vi "Eagle Command Stream Server.vi"(9 "RT Status":refnum<vi>, 10 "StatusRefs":T1, 11 "Controller IP":string="192.168.1.199") -> ()   [LabVIEW 2015]
uses:
  Controls/RT Status Refs.ctl
  Controls/LP Status typedef.ctl
  Controls/BELKIN RT State.ctl
  IP Dev Area/IP results.ctl
  Robo Team Engine Command.ctl
  RT Controls/Generic instruction typedef.ctl
  RT Controls/RT Streamer Ack element.ctl
  Controls/Eagle Green Cordinates.ctl
  <vilib>/vision/Image Controls.llb/IMAQ Image.ctl
  <vilib>/dex/Flush And Wait Empty Condition.ctl
  Controls/Command Typedef.ctl
  Robo Team Globals.vi
  GUI/Host Globals.vi
  <resource>/objmgr/ni.dex.rc
panel:
  out "XY Graph":cluster{"X Cord":u16[], "Y Cord":u16[]}(graph)
  out "Close":bool
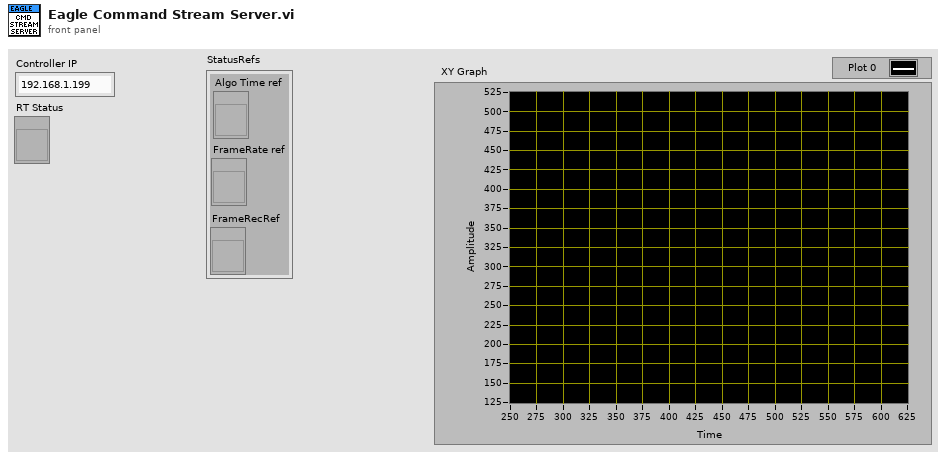
[diagram p1: front panel]
types:
  T1 = typedef "RT Status Refs.ctl" = cluster{"Algo Time ref":refnum<vi>, "FrameRate ref":refnum<vi>, "FrameRecRef":refnum<vi>}
  T2 = typedef "Generic instruction typedef.ctl" = cluster{"CMD":string, "Data":variant}
  T3 = typedef "Robo Team Engine Command.ctl" = cluster{"Command":string, "Data":variant, "Error":errorcluster, "Timeout":i32}
  T4 = typedef "Eagle Green Cordinates.ctl" = cluster{"X Cord":u16[], "Y Cord":u16[]}
  T5 = typedef "LP Status typedef.ctl" = cluster{"FrameRate":dbl, "AlgoTime":dbl, "FrameRec":u16, "System State":T6, "IP Results":T7, "SimulationMode":bool, "RotateImage":bool}
  T6 = typedef "BELKIN RT State.ctl" = enum16{"Initialize", "BIT", "Warm Up", "Eye Location", "Find Limbus", "Eye Track", "Fire", "Treatment Complete", "Shut Down", "Error"}
  T7 = typedef "IP results.ctl" = cluster{"X":u16, "Y":u16, "A":dbl, "B":dbl, "Grade":u16, "Frame#":u16}
  T8 = typedef "RT Streamer Ack element.ctl" = cluster{"Data":variant, "CMD":string, "error":errorcluster}
  T9 = typedef "IMAQ Image.ctl" = refnum<image>
  T10 = typedef "Command Typedef.ctl" = cluster{"CMD":T6, "Data":variant}
  T11 = typedef "Robo System State Refs.ctl" = cluster{"Engage Motor":refnum<vi>, "Auto Level":refnum<vi>, "IMU led":refnum<vi>, "Evaluate Enable":refnum<vi>, "Motor Led":refnum<vi>, "Error Descript":refnum<vi>, "Error Led":refnum<vi>, "Error":refnum<vi>}
  T12 = typedef "Flush And Wait Empty Condition.ctl" = u8
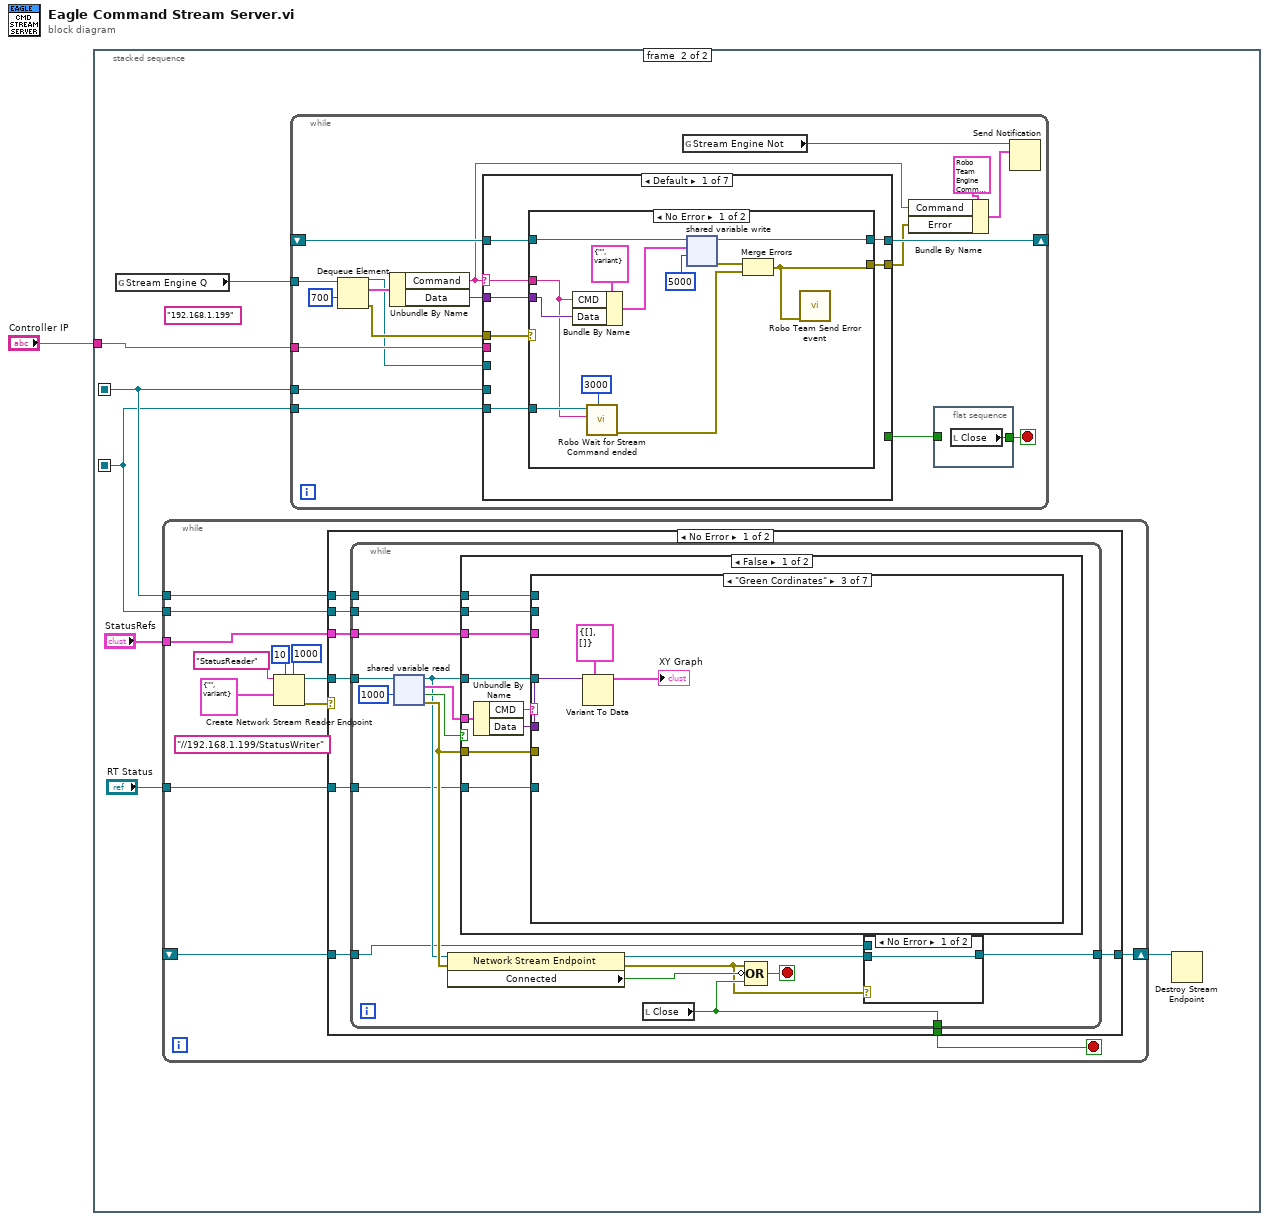
[diagram p0: block diagram]
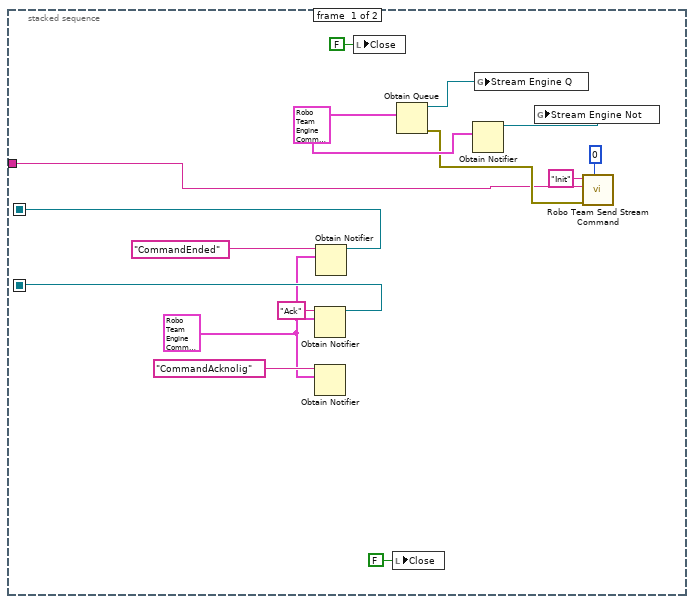
[diagram p2: hidden frame]
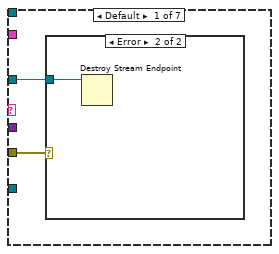
[diagram p4: hidden frame]
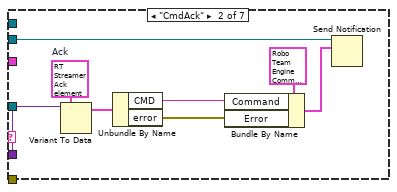
[diagram p6: hidden frame]
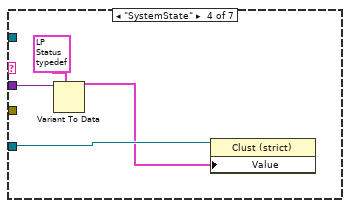
[diagram p7: hidden frame]
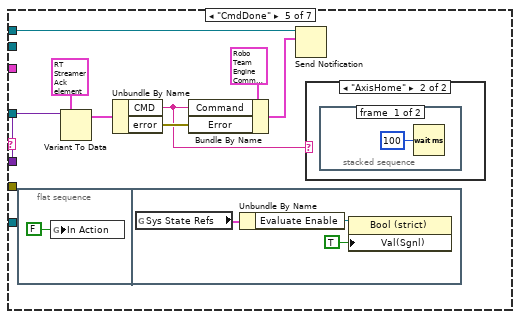
[diagram p8: hidden frame]
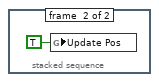
[diagram p10: hidden frame]
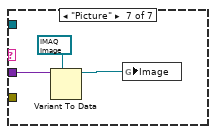
[diagram p12: hidden frame]
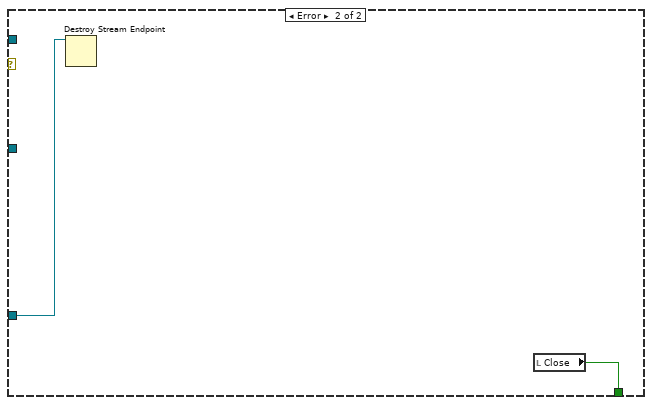
[diagram p14: hidden frame]
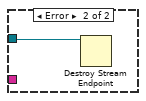
[diagram p15: hidden frame]
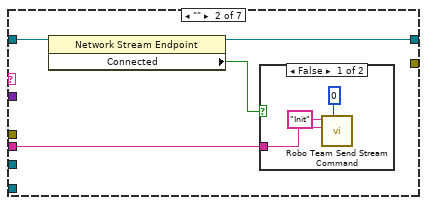
[diagram p16: hidden frame]
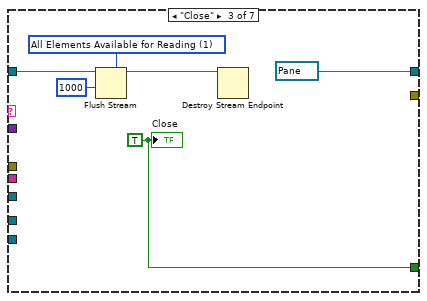
[diagram p18: hidden frame]
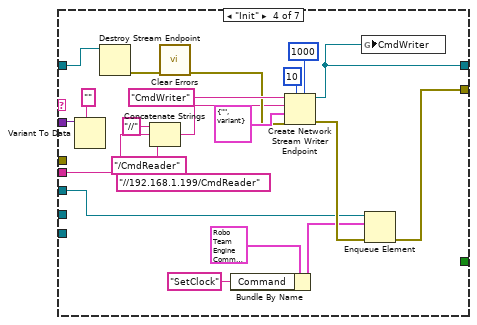
[diagram p19: hidden frame]
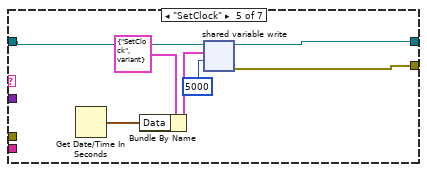
[diagram p20: hidden frame]
diagram:
  n1 = stacked-sequence {
    seq-local: [w14 _] -> [_ w22]
    seq-local: [w12 _] -> [_ w21]
    tunnel: "Controller IP" -> [w2 w18]
    frame #0 {
      w8 = T3 {"Command"="", "Data"=variant, "Error"={"status"=FALSE, "code"=0, "source"=""}, "Timeout"=0} ("notification")
      w11 = T3 {"Command"="", "Data"=variant, "Error"={"status"=FALSE, "code"=0, "source"=""}, "Timeout"=0}
      n2 = Obtain Notifier(name (unnamed)="Ack", notification data type=w11) -> (notifier out=w12:refnum<notifier>)  [unwired: 2 in, 2 out]
      n3 = Obtain Notifier(name (unnamed)="CommandAcknolig", notification data type=w11) -> ()  [unwired: 2 in, 3 out]
      n4 = Obtain Notifier(name (unnamed)="CommandEnded", notification data type=w11) -> (notifier out=w14:refnum<notifier>)  [unwired: 2 in, 2 out]
      n5 = local write "Close"(FALSE ("Close")) -> ()
      n6 = local write "Close"(FALSE ("Close")) -> ()
      n7 = Obtain Queue(element data type=w8) -> (queue out=w7:refnum<queue>, error out=w3:errorcluster)  [unwired: 4 in, 1 out]
      n8 = Obtain Notifier(notification data type=w8) -> (notifier out=w6:refnum<notifier>)  [unwired: 3 in, 2 out]
      n9 = global write "Robo Team Globals.vi" "Stream Engine Q"(w7) -> ()
      n10 = global write "Robo Team Globals.vi" "Stream Engine Not"(w6) -> ()
      n11 = call "Robo Team Send Stream Command.vi"("timeout in ms (0)"=0 ("timeout in ms (5000)"), "error in (no error)"=w3, "Data in"=w2, "Command"="Init") -> ()  [unwired: 6 in, 2 out]
    }
    frame #1 {
      (unwired) "192.168.1.199" ("Controller IP")
      n12 = global read "Robo Team Globals.vi" "Stream Engine Q"() -> (w23:refnum<queue>)
      n13 = while {
        tunnel: w22 -> [w31]
        tunnel: w21 -> [w29]
        shift-right: [w27] -> w19
        shift-left: _ -> [w26]
        tunnel: "StatusRefs" -> [w25]
        tunnel: "RT Status" -> [w24]
        stop <- w30 stop-if-true
        (unwired) "//192.168.1.199/StatusWriter" ("Controller IP")
        n14 = Create Network Stream Reader Endpoint(5:1000 ("timeout in ms (-1)"), 7:10 ("reader buffer size"), 9:T2 {"CMD"="", "Data"=variant}, 11:"StatusReader" ("name (unnamed)")) -> (0:w28:errorcluster, 3:w34:refnum<k21>)  [unwired: 3 in]
        n15 = case shown="No Error" w28 {
          tunnel: w34 -> [w44 _]
          tunnel: w31 -> [w43 _]
          tunnel: [w42 w109] -> w30
          tunnel: w29 -> [w41 _]
          tunnel: [w40 _] -> w27
          tunnel: w26 -> [w39 w108]
          tunnel: w25 -> [w38 _]
          tunnel: w24 -> [w37 _]
          frame No Error {
            n16 = while {
              tunnel: w44 -> [w58]
              tunnel: w43 -> [w56]
              tunnel: [w55] -> w42
              tunnel: w41 -> [w54]
              tunnel: [w48] -> w40
              tunnel: w39 -> [w47]
              tunnel: w38 -> [w46]
              tunnel: w37 -> [w45]
              stop <- w59 stop-if-true
              n17 = shared-variable-read(w58, 1000 ("timeout ms (-1)")) -> (w51:refnum<k21>, w53:errorcluster, w60:bool, w61:T2)  [unwired: 1 in]
              n18 = property class="Network Stream Endpoint"(reference=w51, error in=w53) -> (reference out=w49:refnum<k21>, error out=w50:errorcluster, "Connected"=w52:bool)
              n19 = case shown="False" w60 {
                tunnel: w61 -> [w72 _]
                tunnel: w53 -> [w69 _]
                tunnel: w51 -> [w68 _]
                tunnel: w56 -> [w67 _]
                tunnel: w54 -> [w66 _]
                tunnel: w46 -> [w65 _]
                tunnel: w45 -> [w64 _]
                frame False {
                  n20 = Unbundle By Name(w72) -> ("CMD"=w71:string, "Data"=w70:variant)
                  n21 = case shown="\"Green Cordinates\"" w71 {
                    tunnel: w70 -> [_ w83 w86 w90 w98 _ w107]
                    tunnel: w69 -> [w74 _ _ _ _ _ _]
                    tunnel: w68 -> [w73 _ _ _ _ _ _]
                    tunnel: w67 -> [_ _ _ _ w93 _ _]
                    tunnel: w66 -> [_ w76 _ _ _ _ _]
                    tunnel: w65 -> [_ _ _ _ _ _ _]
                    tunnel: w64 -> [_ _ _ w88 _ _ _]
                    frame Default {
                      n22 = case shown="Error" w74 {
                        tunnel: w73 -> [_ w75]
                        frame No Error {
                        }
                        frame Error {
                          n23 = Destroy Stream Endpoint(11:w75) -> ()  [unwired: 1 in, 1 out]
                        }
                      }
                    }
                    frame "CmdAck" {
                      w82 = T8 {"Data"=variant, "CMD"="", "error"={"status"=FALSE, "code"=0, "source"=""}}  # Ack
                      n24 = Variant To Data(type=w82, Variant=w83) -> (data=w81:T8)  [unwired: 1 in, 1 out]
                      n25 = Unbundle By Name(w81) -> ("CMD"=w78:string, "error"=w77:errorcluster)
                      n26 = Bundle By Name(cluster=T3 {"Command"="", "Data"=variant, "Error"={"status"=FALSE, "code"=0, "source"=""}, "Timeout"=0} ("element"), "Command"=w78, "Error"=w77) -> (w79:T3)
                      n27 = Send Notification(notification=w79, notifier=w76) -> ()  [unwired: 1 in, 2 out]
                    }
                    frame "Green Cordinates" {
                      n28 = Variant To Data(type=T4 {"X Cord"=[], "Y Cord"=[]}, Variant=w86) -> (data=→"XY Graph":T4)  [unwired: 1 in, 1 out]
                    }
                    frame "SystemState" {
                      n29 = Variant To Data(type=T5 {"FrameRate"=0.0, "AlgoTime"=0.0, "FrameRec"=0, "System State"=enum."Find Limbus", "IP Results"={"X"=0, "Y"=0, "A"=0.0, "B"=0.0, "Grade"=0, "Frame#"=0}, "SimulationMode"=FALSE, "RotateImage"=FALSE} ("LP Status"), Variant=w90) -> (data=w87:T5)  [unwired: 1 in, 1 out]
                      n30 = property class="Clust (strict)"(reference=w88, "Value"=w87) -> ()  [unwired: 1 in, 2 out]
                    }
                    frame "CmdDone" {
                      n31 = flat-sequence {
                        frame #0 {
                          n32 = global write "Robo Team Globals.vi" "In Action"(FALSE ("In Action")) -> ()
                        }
                        frame #1 {
                          n33 = global read "Robo Team Globals.vi" "Sys State Refs"() -> (w102:T11)
                          n34 = Unbundle By Name(w102) -> ("Evaluate Enable"=w103:refnum<vi>)
                          n35 = property class="Bool (strict)"(reference=w103, "Val(Sgnl)"=TRUE ("Value (Signaling)")) -> ()  [unwired: 1 in, 2 out]
                        }
                      }
                      n36 = Variant To Data(type=T8 {"Data"=variant, "CMD"="", "error"={"status"=FALSE, "code"=0, "source"=""}} ("Ack"), Variant=w98) -> (data=w96:T8)  [unwired: 1 in, 1 out]
                      n37 = Unbundle By Name(w96) -> ("CMD"=w91:string, "error"=w94:errorcluster)
                      n38 = Bundle By Name(cluster=T3 {"Command"="", "Data"=variant, "Error"={"status"=FALSE, "code"=0, "source"=""}, "Timeout"=0} ("element"), "Command"=w91, "Error"=w94) -> (w92:T3)
                      n39 = Send Notification(notification=w92, notifier=w93) -> ()  [unwired: 1 in, 2 out]
                      n40 = case shown="\"AxisHome\"" w91 {
                        frame Default {
                        }
                        frame "AxisHome" {
                          n41 = stacked-sequence {
                            frame #0 {
                              n42 = Wait (ms)(milliseconds to wait=u32 100) -> ()  [unwired: 1 out]
                            }
                            frame #1 {
                              n43 = global write "Robo Team Globals.vi" "Update Pos"(TRUE ("Update Pos")) -> ()
                            }
                          }
                        }
                      }
                    }
                    frame "Status" {
                    }
                    frame "Picture" {
                      n44 = Variant To Data(type=T9 refnum ("Image"), Variant=w107) -> (data=w105:T9)  [unwired: 1 in, 1 out]
                      n45 = global write "Host Globals.vi" "Image"(w105) -> ()
                    }
                  }
                }
                frame True {
                }
              }
              n46 = local read "Close"() -> (w55:bool)
              n47 = Compound Arithmetic op=OR(w50, invert w52, w55) -> (w59:bool)
              n48 = case shown="No Error" w50 {
                tunnel: [w62 w63] -> w48
                tunnel: w49 -> [w62 _]
                tunnel: w47 -> [_ w63]
                frame No Error {
                }
                frame Error {
                }
              }
            }
          }
          frame Error {
            n49 = Destroy Stream Endpoint(11:w108) -> ()  [unwired: 1 in, 1 out]
            n50 = local read "Close"() -> (w109:bool)
          }
        }
      }
      n51 = while {
        tunnel: w23 -> [w127]
        shift-right: [w124] -> _
        shift-left: _ -> [w123]
        tunnel: w22 -> [w115]
        tunnel: w21 -> [w113]
        tunnel: w18 -> [w111]
        stop <- w116 stop-if-true
        n52 = Dequeue Element(queue=w127, timeout in ms (-1)=700) -> (queue out=w110:refnum<queue>, element=w126:T3, error out=w122:errorcluster)  [unwired: 1 in, 1 out]
        n53 = Unbundle By Name(w126) -> ("Command"=w118:string, "Data"=w125:variant)
        n54 = case shown="Default" w118 {
          selector: w118 -> [w132 _ _ _ _ _ _]
          tunnel: w125 -> [w131 _ _ w178 _ w190 w200]
          tunnel: [w133 w151 refnum<k21> refnum ("writer name") w170 w186 w195 w204] -> w124
          tunnel: w123 -> [w134 w152 w161 w174 w187 w196 w205]
          tunnel: w122 -> [w135 _ _ _ _ _ _]
          tunnel: [w129 _ _ w168 w182 w194 w203] -> w117
          tunnel: w115 -> [_ _ _ _ _ _ _]
          tunnel: [_ _ w159 _ _ _ _] -> w114
          tunnel: w113 -> [w130 _ _ _ _ _ _]
          tunnel: w111 -> [_ w149 _ w163 _ _ _]
          tunnel: w110 -> [_ _ _ w167 _ _ _]
          frame Default {
            n55 = case shown="No Error" w135 {
              tunnel: w134 -> [w146 w148]
              tunnel: [w145 _] -> w133
              tunnel: w132 -> [w140 _]
              tunnel: w131 -> [w142 _]
              tunnel: w130 -> [w141 _]
              tunnel: [w137 _] -> w129
              frame No Error {
                n56 = Bundle By Name(cluster=T2 {"CMD"="", "Data"=variant} ("data in"), "CMD"=w140, "Data"=w142) -> (w143:T2)
                n57 = call "Robo Wait for Stream Command ended.vi"("Timeout"=u32 3000, "Command"=w140, "Notifier in"=w141) -> ("error out"=w138:errorcluster)  [unwired: 8 in]
                n58 = shared-variable-write(w146, w143, 5000 ("timeout ms (-1)")) -> (w145:refnum<k21>, w139:errorcluster)  [unwired: 1 in, 1 out]
                n59 = Merge Errors(w139, w138) -> (w137:errorcluster)
                n60 = call "Robo Team Send Error event.vi"("error in (no error)"=w137) -> ()  [unwired: 11 in]
              }
              frame Error {
                n61 = Destroy Stream Endpoint(11:w148) -> ()  [unwired: 1 in, 1 out]
              }
            }
          }
          frame "" {
            n62 = property class="Network Stream Endpoint"(reference=w152) -> (reference out=w151:refnum<k21>, "Connected"=w150:bool)  [unwired: 1 in, 1 out]
            n63 = case shown="False" w150 {
              tunnel: w149 -> [w153 _]
              frame False {
                n64 = call "Robo Team Send Stream Command.vi"("timeout in ms (0)"=0 ("timeout in ms (5000)"), "Data in"=w153, "Command"="Init") -> ()  [unwired: 7 in, 2 out]
              }
              frame True {
              }
            }
          }
          frame "Close" {
            w157 = T12 1 items=["All Elements Read From Stream", "All Elements Available for Reading"] ("wait condition")
            w159 = TRUE ("Close")
            n65 = Flush Stream(9:1000 ("timeout in ms (-1)"), 10:w157, 11:w161) -> (3:w158:refnum<k21>)  [unwired: 1 in, 2 out]
            n66 = Destroy Stream Endpoint(11:w158) -> ()  [unwired: 1 in, 1 out]
            "Close" <- w159
          }
          frame "Init" {
            (unwired) "//192.168.1.199/CmdReader" ("Controller IP")
            n67 = Variant To Data(type="", Variant=w178) -> ()  [unwired: 1 in, 2 out]
            n68 = Destroy Stream Endpoint(11:w174) -> (0:w173:errorcluster)  [unwired: 1 in]
            n69 = Concatenate Strings("//" ("string"), w163, "/CmdReader" ("string")) -> (w162:string)
            n70 = call <vilib>:"Clear Errors.vi"("error in (no error)"=w173) -> ("error out"=w172:errorcluster)  [unwired: 5 in, 1 out]
            n71 = Bundle By Name(cluster=T3 {"Command"="", "Data"=variant, "Error"={"status"=FALSE, "code"=0, "source"=""}, "Timeout"=0} ("element"), "Command"="SetClock") -> (w165:T3)
            n72 = Create Network Stream Writer Endpoint(5:1000 ("timeout in ms (-1)"), 7:10 ("writer buffer size"), 8:w172, 9:T2 {"CMD"="", "Data"=variant}, 10:w162, 11:"CmdWriter" ("writer name")) -> (0:w169:errorcluster, 3:w170:refnum<k21>)  [unwired: 1 in]
            n73 = global write "Robo Team Globals.vi" "CmdWriter"(w170) -> ()
            n74 = Enqueue Element(queue=w167, element=w165, error in (no error)=w169) -> (error out=w168:errorcluster)  [unwired: 1 in, 2 out]
          }
          frame "SetClock" {
            n75 = Get Date/Time In Seconds() -> (seconds since 1Jan1904=w183:timestamp)
            n76 = Bundle By Name(cluster=T2 {"CMD"="SetClock", "Data"=variant} ("data in"), "Data"=w183) -> (w184:T2)
            n77 = shared-variable-write(w187, w184, 5000 ("timeout ms (-1)")) -> (w186:refnum<k21>, w182:errorcluster)  [unwired: 1 in, 1 out]
          }
          frame "SetSystemState" {
            n78 = Variant To Data(type=T10 {"CMD"=enum."Find Limbus", "Data"=variant} ("element"), Variant=w190) -> (data=w189:T10)  [unwired: 1 in, 1 out]
            n79 = Bundle By Name(cluster=T2 {"CMD"="SetSystemState", "Data"=variant} ("data in"), "Data"=w189) -> (w192:T2)
            n80 = shared-variable-write(w196, w192, 5000 ("timeout ms (-1)")) -> (w195:refnum<k21>, w194:errorcluster)  [unwired: 1 in, 1 out]
          }
          frame "SetSimulationMode" {
            n81 = Variant To Data(type=TRUE, Variant=w200) -> (data=w199:bool)  [unwired: 1 in, 1 out]
            n82 = Bundle By Name(cluster=T2 {"CMD"="SetSimulationMode", "Data"=variant} ("data in"), "Data"=w199) -> (w201:T2)
            n83 = shared-variable-write(w205, w201, 5000 ("timeout ms (-1)")) -> (w204:refnum<k21>, w203:errorcluster)  [unwired: 1 in, 1 out]
          }
        }
        n84 = global read "Robo Team Globals.vi" "Stream Engine Not"() -> (w121:refnum<notifier>)
        n85 = Bundle By Name(cluster=T3 {"Command"="", "Data"=variant, "Error"={"status"=FALSE, "code"=0, "source"=""}, "Timeout"=0} ("notification"), "Command"=w118, "Error"=w117) -> (w120:T3)
        n86 = flat-sequence {
          tunnel: [w128] -> w116
          tunnel: w114 -> [_]
          frame #0 {
            n87 = local read "Close"() -> (w128:bool)
          }
        }
        n88 = Send Notification(notification=w120, notifier=w121) -> ()  [unwired: 1 in, 2 out]
      }
      n89 = Destroy Stream Endpoint(11:w19) -> ()  [unwired: 1 in, 1 out]
    }
  }
